vi "Nahum_spaceapps.vi"() -> ()   [LabVIEW 2013]
uses:
  <vilib>/Analysis/Matrix/Datatypes/RealMatrix.ctl
  <vilib>/Analysis/Matrix/Numeric/Conversions/Array To Matrix - RA2.vi
  <vilib>/Analysis/Matrix/NI_Matrix.lvlib
panel:
  out "Presion arterial":string
  out "RADIACIÓN AREA":string
  out "RC.PERSONA":string
  out "TEMP.AREA":string
  out "RADIACION EEI":string
  out "TEMP. PERSONA":string
  out "HUMEDAD AREA":string
  out "OXIGENO AREA":string
  out "VELOCIDAD EEI":string
  out "LATITUD EEI":string
  out "PRESIÓN AREA":string
  out "ILUMINACIÓN AREA":string
  out "ALTITUD EEI":string
  out "LONGITUD EEI":string
  out "GRAVEDAD AREA":string
  out "OXIGENO PERSONA":string
  out "ENERGIA":string
  out "GRAVEDAD AREA":dbl
  out "LATITUD EEI":dbl
  out "RADIACION AREA":dbl
  out "ILUMINACION AREA":dbl
  out "HUMEDAD AREA":dbl
  out "OXIGENO AREA":dbl
  out "PRESION AREA":dbl
  out "TEMP. AREA":dbl
  out "OXIGENO PERSONA":dbl
  out "RC. PERSONA":dbl
  out "PA.PERSONA":dbl
  out "TEMP.PERSONA":dbl
  out "LONGITUD EEI":dbl
  out "ALTITUD EEI":dbl
  out "VELOCIDAD EEI":dbl
  out "RADIACION EEI":dbl
  out "ENERGIA":dbl
  out "ENERGIA":T1
  out "ENERGIA":dbl[][](array[numeric])
  out "RADIACION EEI":T1
  out "RADIACION EEI":dbl[][](array[numeric])
  out "VELOCIDAD EEI":T1
  out "VELOCIDAD EEI":dbl[][](array[numeric])
  out "ALTITUD EEI":T1
  out "ALTITUD EEI":dbl[][](array[numeric])
  out "LONGITUD EEI":T1
  out "LONGITUD EEI":dbl[][](array[numeric])
  out "LATITUD EEI":T1
  out "LATITUD EEI":dbl[][](array[numeric])
  out "ILUMINACION AREA":T1
  out "ILUMINACION AREA":dbl[][](array[numeric])
  out "GRAVEDAD AREA":T1
  out "GRAVEDAD AREA":dbl[][](array[numeric])
  out "HUMEDAD AREA":T1
  out "HUMEDAD AREA":dbl[][](array[numeric])
  out "RADIACION AREA":T1
  out "RADIACION AREA":dbl[][](array[numeric])
  out "OXIGENO AREA":T1
  out "OXIGENO AREA":dbl[][](array[numeric])
  out "PRESION AREA":T1
  out "PRESION AREA":dbl[][](array[numeric])
  out "TEMP. AREA":T1
  out "TEMP. AREA":dbl[][](array[numeric])
  out "Oxigeno PERSONA":T1
  out "Oxigeno SANGRE PERSONA":dbl[][](array[numeric])
  out "RC. PERSONA":T1
  out "Ritmo Cardiaco":dbl[][](array[numeric])
  out "PA. PERSONA":T1
  out "PRESION ARTERIAL PERSONA":dbl[][](array[numeric])
  out "TEMP.PERSONA":T1
  out "TEMP.PERSONA":dbl[][](array[numeric])
  out "R10":dbl
  out "R9":dbl
  out "R8":dbl
  out "R7":dbl
  out "R6":dbl
  out "R5":dbl
  out "R4":dbl
  out "R3":dbl
  out "R2":dbl
  in  "stop":bool
  out "R1":dbl
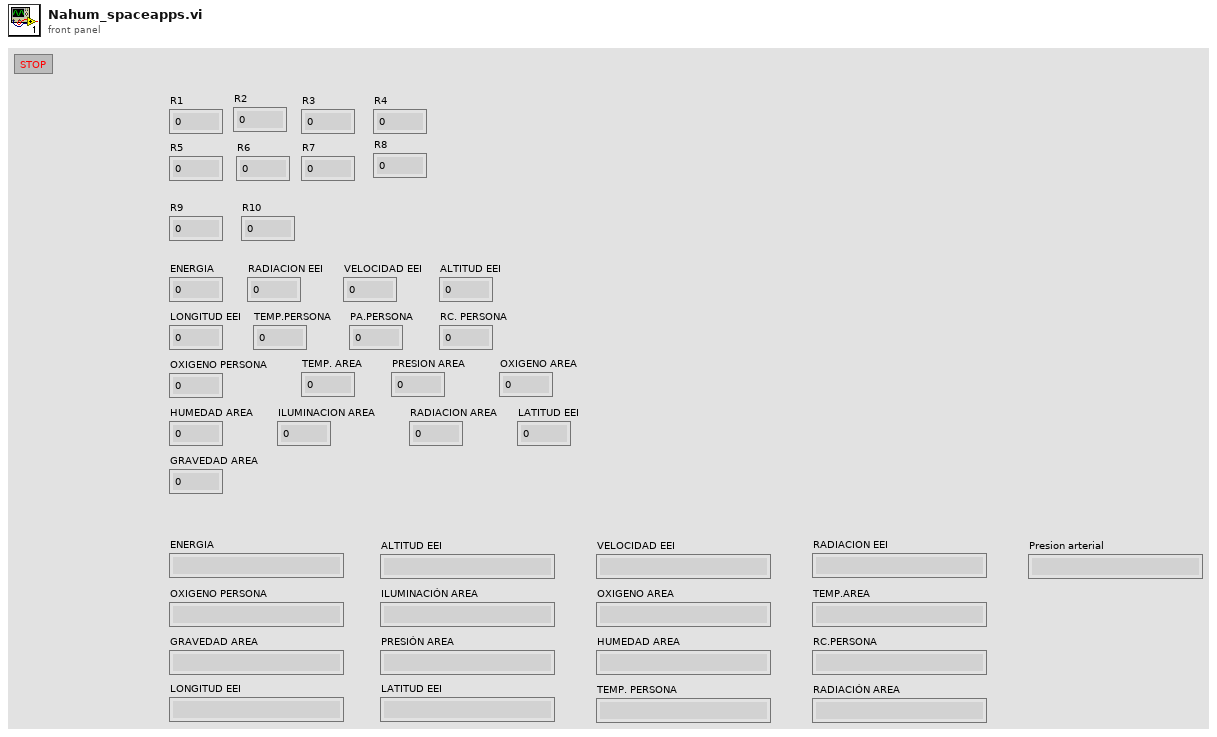
[diagram p1: front panel]
types:
  T1 = typedef "NI_Matrix.lvlib/RealMatrix.ctl" = dbl[][]
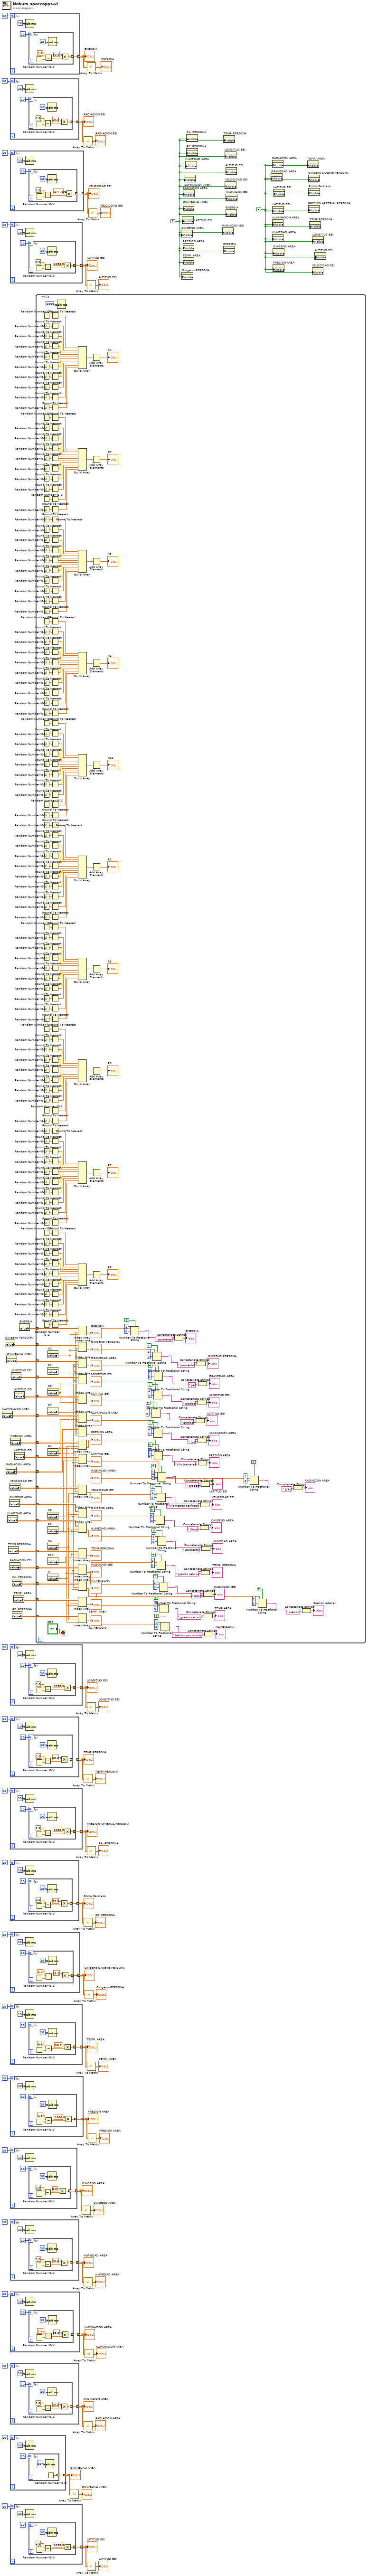
[diagram p0: block diagram]
diagram:
  w2 = FALSE
  w1 = FALSE
  n1 = property on="ILUMINACION AREA" class="Arr (strict)"() -> ("Value"=w6:T1)  [unwired: 2 in, 2 out]
  n2 = property on="Oxigeno PERSONA" class="Arr (strict)"() -> ("Value"=w11:T1)  [unwired: 2 in, 2 out]
  n3 = property on="RADIACION AREA" class="Arr (strict)"() -> ("Value"=w5:T1)  [unwired: 2 in, 2 out]
  n4 = property on="GRAVEDAD AREA" class="Arr (strict)"() -> ("Value"=w3:T1)  [unwired: 2 in, 2 out]
  n5 = property on="HUMEDAD AREA" class="Arr (strict)"() -> ("Value"=w7:T1)  [unwired: 2 in, 2 out]
  n6 = property on="TEMP.PERSONA" class="Arr (strict)"() -> ("Value"=w14:T1)  [unwired: 2 in, 2 out]
  n7 = property on="OXIGENO AREA" class="Arr (strict)"() -> ("Value"=w8:T1)  [unwired: 2 in, 2 out]
  n8 = property on="VELOCIDAD EEI" class="Arr (strict)"() -> ("Value"=w17:T1)  [unwired: 2 in, 2 out]
  n9 = property on="RADIACION EEI" class="Arr (strict)"() -> ("Value"=w18:T1)  [unwired: 2 in, 2 out]
  n10 = for {
    N: 10 -> [_]
    tunnel: [w73] -> w22 mode=indexing
    n11 = Wait (ms)(milliseconds to wait=u32 10) -> ()  [unwired: 1 out]
    n12 = for {
      N: 10 -> [_]
      tunnel: [w74] -> w73 mode=indexing
      n13 = Random Number (0-1)() -> (number: 0 to 1=w77:dbl)
      n14 = Subtract(x=1.8, y=w77) -> (x-y=w76:dbl)
      n15 = Wait (ms)(milliseconds to wait=u32 10) -> ()  [unwired: 1 out]
      n16 = Multiply(x=80.0, y=w76) -> (x*y=w74:dbl)
    }
  }
  "ENERGIA" <- w22
  n17 = for {
    N: 10 -> [_]
    tunnel: [w82] -> w25 mode=indexing
    n18 = Wait (ms)(milliseconds to wait=u32 10) -> ()  [unwired: 1 out]
    n19 = for {
      N: 10 -> [_]
      tunnel: [w83] -> w82 mode=indexing
      n20 = Random Number (0-1)() -> (number: 0 to 1=w86:dbl)
      n21 = Subtract(x=1.0, y=w86) -> (x-y=w85:dbl)
      n22 = Wait (ms)(milliseconds to wait=u32 10) -> ()  [unwired: 1 out]
      n23 = Multiply(x=10.0, y=w85) -> (x*y=w83:dbl)
    }
  }
  "RADIACION EEI" <- w25
  n24 = for {
    N: 10 -> [_]
    tunnel: [w91] -> w28 mode=indexing
    n25 = Wait (ms)(milliseconds to wait=u32 10) -> ()  [unwired: 1 out]
    n26 = for {
      N: 10 -> [_]
      tunnel: [w92] -> w91 mode=indexing
      n27 = Random Number (0-1)() -> (number: 0 to 1=w95:dbl)
      n28 = Subtract(x=2.0, y=w95) -> (x-y=w94:dbl)
      n29 = Wait (ms)(milliseconds to wait=u32 10) -> ()  [unwired: 1 out]
      n30 = Multiply(x=27743.0, y=w94) -> (x*y=w92:dbl)
    }
  }
  "VELOCIDAD EEI" <- w28
  n31 = for {
    N: 10 -> [_]
    tunnel: [w100] -> w31 mode=indexing
    n32 = Wait (ms)(milliseconds to wait=u32 10) -> ()  [unwired: 1 out]
    n33 = for {
      N: 10 -> [_]
      tunnel: [w101] -> w100 mode=indexing
      n34 = Random Number (0-1)() -> (number: 0 to 1=w104:dbl)
      n35 = Subtract(x=2.0, y=w104) -> (x-y=w103:dbl)
      n36 = Wait (ms)(milliseconds to wait=u32 10) -> ()  [unwired: 1 out]
      n37 = Multiply(x=1250.0, y=w103) -> (x*y=w101:dbl)
    }
  }
  "ALTITUD EEI" <- w31
  n38 = for {
    N: 10 -> [_]
    tunnel: [w109] -> w34 mode=indexing
    n39 = Wait (ms)(milliseconds to wait=u32 10) -> ()  [unwired: 1 out]
    n40 = for {
      N: 10 -> [_]
      tunnel: [w110] -> w109 mode=indexing
      n41 = Random Number (0-1)() -> (number: 0 to 1=w113:dbl)
      n42 = Subtract(x=2.0, y=w113) -> (x-y=w112:dbl)
      n43 = Wait (ms)(milliseconds to wait=u32 10) -> ()  [unwired: 1 out]
      n44 = Multiply(x=1250.0, y=w112) -> (x*y=w110:dbl)
    }
  }
  "LONGITUD EEI" <- w34
  n45 = for {
    N: 10 -> [_]
    tunnel: [w118] -> w70 mode=indexing
    n46 = Wait (ms)(milliseconds to wait=u32 10) -> ()  [unwired: 1 out]
    n47 = for {
      N: 10 -> [_]
      tunnel: [w119] -> w118 mode=indexing
      n48 = Random Number (0-1)() -> (number: 0 to 1=w122:dbl)
      n49 = Subtract(x=2.0, y=w122) -> (x-y=w121:dbl)
      n50 = Wait (ms)(milliseconds to wait=u32 10) -> ()  [unwired: 1 out]
      n51 = Multiply(x=29.0, y=w121) -> (x*y=w119:dbl)
    }
  }
  "TEMP.PERSONA" <- w70
  n52 = for {
    N: 10 -> [_]
    tunnel: [w127] -> w68 mode=indexing
    n53 = Wait (ms)(milliseconds to wait=u32 10) -> ()  [unwired: 1 out]
    n54 = for {
      N: 10 -> [_]
      tunnel: [w128] -> w127 mode=indexing
      n55 = Random Number (0-1)() -> (number: 0 to 1=w131:dbl)
      n56 = Subtract(x=2.0, y=w131) -> (x-y=w130:dbl)
      n57 = Wait (ms)(milliseconds to wait=u32 10) -> ()  [unwired: 1 out]
      n58 = Multiply(x=1250.0, y=w130) -> (x*y=w128:dbl)
    }
  }
  "PRESION ARTERIAL PERSONA" <- w68
  n59 = for {
    N: 10 -> [_]
    tunnel: [w136] -> w64 mode=indexing
    n60 = Wait (ms)(milliseconds to wait=u32 10) -> ()  [unwired: 1 out]
    n61 = for {
      N: 10 -> [_]
      tunnel: [w137] -> w136 mode=indexing
      n62 = Random Number (0-1)() -> (number: 0 to 1=w140:dbl)
      n63 = Subtract(x=2.0, y=w140) -> (x-y=w139:dbl)
      n64 = Wait (ms)(milliseconds to wait=u32 10) -> ()  [unwired: 1 out]
      n65 = Multiply(x=55.0, y=w139) -> (x*y=w137:dbl)
    }
  }
  "Ritmo Cardiaco" <- w64
  n66 = for {
    N: 10 -> [_]
    tunnel: [w145] -> w62 mode=indexing
    n67 = Wait (ms)(milliseconds to wait=u32 10) -> ()  [unwired: 1 out]
    n68 = for {
      N: 10 -> [_]
      tunnel: [w146] -> w145 mode=indexing
      n69 = Random Number (0-1)() -> (number: 0 to 1=w149:dbl)
      n70 = Subtract(x=1.4, y=w149) -> (x-y=w148:dbl)
      n71 = Wait (ms)(milliseconds to wait=u32 10) -> ()  [unwired: 1 out]
      n72 = Multiply(x=95.0, y=w148) -> (x*y=w146:dbl)
    }
  }
  "Oxigeno SANGRE PERSONA" <- w62
  n73 = for {
    N: 10 -> [_]
    tunnel: [w154] -> w58 mode=indexing
    n74 = Wait (ms)(milliseconds to wait=u32 10) -> ()  [unwired: 1 out]
    n75 = for {
      N: 10 -> [_]
      tunnel: [w155] -> w154 mode=indexing
      n76 = Random Number (0-1)() -> (number: 0 to 1=w158:dbl)
      n77 = Subtract(x=1.6, y=w158) -> (x-y=w157:dbl)
      n78 = Wait (ms)(milliseconds to wait=u32 10) -> ()  [unwired: 1 out]
      n79 = Multiply(x=26.5, y=w157) -> (x*y=w155:dbl)
    }
  }
  "TEMP. AREA" <- w58
  n80 = for {
    N: 10 -> [_]
    tunnel: [w163] -> w55 mode=indexing
    n81 = Wait (ms)(milliseconds to wait=u32 10) -> ()  [unwired: 1 out]
    n82 = for {
      N: 10 -> [_]
      tunnel: [w164] -> w163 mode=indexing
      n83 = Random Number (0-1)() -> (number: 0 to 1=w167:dbl)
      n84 = Subtract(x=1.5, y=w167) -> (x-y=w166:dbl)
      n85 = Wait (ms)(milliseconds to wait=u32 10) -> ()  [unwired: 1 out]
      n86 = Multiply(x=1000.0, y=w166) -> (x*y=w164:dbl)
    }
  }
  "PRESION AREA" <- w55
  n87 = for {
    N: 10 -> [_]
    tunnel: [w172] -> w52 mode=indexing
    n88 = Wait (ms)(milliseconds to wait=u32 10) -> ()  [unwired: 1 out]
    n89 = for {
      N: 10 -> [_]
      tunnel: [w173] -> w172 mode=indexing
      n90 = Random Number (0-1)() -> (number: 0 to 1=w176:dbl)
      n91 = Subtract(x=2.0, y=w176) -> (x-y=w175:dbl)
      n92 = Wait (ms)(milliseconds to wait=u32 10) -> ()  [unwired: 1 out]
      n93 = Multiply(x=6.0, y=w175) -> (x*y=w173:dbl)
    }
  }
  "OXIGENO AREA" <- w52
  n94 = for {
    N: 10 -> [_]
    tunnel: [w181] -> w46 mode=indexing
    n95 = Wait (ms)(milliseconds to wait=u32 10) -> ()  [unwired: 1 out]
    n96 = for {
      N: 10 -> [_]
      tunnel: [w182] -> w181 mode=indexing
      n97 = Random Number (0-1)() -> (number: 0 to 1=w185:dbl)
      n98 = Subtract(x=2.0, y=w185) -> (x-y=w184:dbl)
      n99 = Wait (ms)(milliseconds to wait=u32 10) -> ()  [unwired: 1 out]
      n100 = Multiply(x=40.0, y=w184) -> (x*y=w182:dbl)
    }
  }
  "HUMEDAD AREA" <- w46
  n101 = for {
    N: 10 -> [_]
    tunnel: [w190] -> w40 mode=indexing
    n102 = Wait (ms)(milliseconds to wait=u32 10) -> ()  [unwired: 1 out]
    n103 = for {
      N: 10 -> [_]
      tunnel: [w191] -> w190 mode=indexing
      n104 = Random Number (0-1)() -> (number: 0 to 1=w194:dbl)
      n105 = Subtract(x=1.4, y=w194) -> (x-y=w193:dbl)
      n106 = Wait (ms)(milliseconds to wait=u32 10) -> ()  [unwired: 1 out]
      n107 = Multiply(x=95.0, y=w193) -> (x*y=w191:dbl)
    }
  }
  "ILUMINACION AREA" <- w40
  n108 = for {
    N: 10 -> [_]
    tunnel: [w199] -> w49 mode=indexing
    n109 = Wait (ms)(milliseconds to wait=u32 10) -> ()  [unwired: 1 out]
    n110 = for {
      N: 10 -> [_]
      tunnel: [w200] -> w199 mode=indexing
      n111 = Random Number (0-1)() -> (number: 0 to 1=w203:dbl)
      n112 = Subtract(x=2.0, y=w203) -> (x-y=w202:dbl)
      n113 = Wait (ms)(milliseconds to wait=u32 10) -> ()  [unwired: 1 out]
      n114 = Multiply(x=10.0, y=w202) -> (x*y=w200:dbl)
    }
  }
  "RADIACION AREA" <- w49
  n115 = for {
    N: 10 -> [_]
    tunnel: [w208] -> w43 mode=indexing
    n116 = Wait (ms)(milliseconds to wait=u32 10) -> ()  [unwired: 1 out]
    n117 = for {
      N: 10 -> [_]
      tunnel: [w209] -> w208 mode=indexing
      n118 = Wait (ms)(milliseconds to wait=u32 10) -> ()  [unwired: 1 out]
      n119 = Random Number (0-1)() -> (number: 0 to 1=w209:dbl)
    }
  }
  "GRAVEDAD AREA" <- w43
  n120 = for {
    N: 10 -> [_]
    tunnel: [w213] -> w37 mode=indexing
    n121 = Wait (ms)(milliseconds to wait=u32 10) -> ()  [unwired: 1 out]
    n122 = for {
      N: 10 -> [_]
      tunnel: [w214] -> w213 mode=indexing
      n123 = Random Number (0-1)() -> (number: 0 to 1=w217:dbl)
      n124 = Subtract(x=2.0, y=w217) -> (x-y=w216:dbl)
      n125 = Wait (ms)(milliseconds to wait=u32 10) -> ()  [unwired: 1 out]
      n126 = Multiply(x=1250.0, y=w216) -> (x*y=w214:dbl)
    }
  }
  "LATITUD EEI" <- w37
  n127 = property on="PRESION AREA" class="Arr (strict)"() -> ("Value"=w9:T1)  [unwired: 2 in, 2 out]
  n128 = property on="LONGITUD EEI" class="Arr (strict)"() -> ("Value"=w15:T1)  [unwired: 2 in, 2 out]
  n129 = property on="PA. PERSONA" class="Arr (strict)"() -> ("Value"=w13:T1)  [unwired: 2 in, 2 out]
  n130 = property on="RC. PERSONA" class="Arr (strict)"() -> ("Value"=w12:T1)  [unwired: 2 in, 2 out]
  n131 = property on="TEMP. AREA" class="Arr (strict)"() -> ("Value"=w10:T1)  [unwired: 2 in, 2 out]
  n132 = property on="ALTITUD EEI" class="Arr (strict)"() -> ("Value"=w16:T1)  [unwired: 2 in, 2 out]
  n133 = property on="LATITUD EEI" class="Arr (strict)"() -> ("Value"=w4:T1)  [unwired: 2 in, 2 out]
  n134 = property on="ENERGIA" class="Arr (strict)"() -> ("Value"=w19:T1)  [unwired: 2 in, 2 out]
  n135 = while {
    tunnel: w19 -> [w365]
    tunnel: w18 -> [w364]
    tunnel: w17 -> [w363]
    tunnel: w16 -> [w362]
    tunnel: w15 -> [w361]
    tunnel: w14 -> [w360]
    tunnel: w13 -> [w359]
    tunnel: w12 -> [w358]
    tunnel: w11 -> [w357]
    tunnel: w10 -> [w356]
    tunnel: w9 -> [w355]
    tunnel: w8 -> [w354]
    tunnel: w7 -> [w353]
    tunnel: w6 -> [w352]
    tunnel: w5 -> [w351]
    tunnel: w4 -> [w350]
    tunnel: w3 -> [w349]
    stop <- "stop" stop-if-true
    n136 = Random Number (0-1)() -> (number: 0 to 1=w500:dbl)
    n137 = Random Number (0-1)() -> (number: 0 to 1=w501:dbl)
    n138 = Random Number (0-1)() -> (number: 0 to 1=w502:dbl)
    n139 = Random Number (0-1)() -> (number: 0 to 1=w503:dbl)
    n140 = Random Number (0-1)() -> (number: 0 to 1=w504:dbl)
    n141 = Random Number (0-1)() -> (number: 0 to 1=w505:dbl)
    n142 = Random Number (0-1)() -> (number: 0 to 1=w506:dbl)
    n143 = Random Number (0-1)() -> (number: 0 to 1=w507:dbl)
    n144 = Random Number (0-1)() -> (number: 0 to 1=w508:dbl)
    n145 = Random Number (0-1)() -> (number: 0 to 1=w509:dbl)
    n146 = Random Number (0-1)() -> (number: 0 to 1=w434:dbl)
    n147 = Random Number (0-1)() -> (number: 0 to 1=w435:dbl)
    n148 = Random Number (0-1)() -> (number: 0 to 1=w436:dbl)
    n149 = Random Number (0-1)() -> (number: 0 to 1=w437:dbl)
    n150 = Random Number (0-1)() -> (number: 0 to 1=w438:dbl)
    n151 = Random Number (0-1)() -> (number: 0 to 1=w439:dbl)
    n152 = Random Number (0-1)() -> (number: 0 to 1=w440:dbl)
    n153 = Random Number (0-1)() -> (number: 0 to 1=w441:dbl)
    n154 = Random Number (0-1)() -> (number: 0 to 1=w442:dbl)
    n155 = Random Number (0-1)() -> (number: 0 to 1=w443:dbl)
    n156 = Random Number (0-1)() -> (number: 0 to 1=w478:dbl)
    n157 = Random Number (0-1)() -> (number: 0 to 1=w479:dbl)
    n158 = Random Number (0-1)() -> (number: 0 to 1=w480:dbl)
    n159 = Random Number (0-1)() -> (number: 0 to 1=w481:dbl)
    n160 = Random Number (0-1)() -> (number: 0 to 1=w482:dbl)
    n161 = Random Number (0-1)() -> (number: 0 to 1=w483:dbl)
    n162 = Random Number (0-1)() -> (number: 0 to 1=w484:dbl)
    n163 = Random Number (0-1)() -> (number: 0 to 1=w485:dbl)
    n164 = Random Number (0-1)() -> (number: 0 to 1=w486:dbl)
    n165 = Random Number (0-1)() -> (number: 0 to 1=w487:dbl)
    n166 = Random Number (0-1)() -> (number: 0 to 1=w456:dbl)
    n167 = Random Number (0-1)() -> (number: 0 to 1=w457:dbl)
    n168 = Random Number (0-1)() -> (number: 0 to 1=w458:dbl)
    n169 = Random Number (0-1)() -> (number: 0 to 1=w459:dbl)
    n170 = Random Number (0-1)() -> (number: 0 to 1=w460:dbl)
    n171 = Random Number (0-1)() -> (number: 0 to 1=w461:dbl)
    n172 = Random Number (0-1)() -> (number: 0 to 1=w462:dbl)
    n173 = Random Number (0-1)() -> (number: 0 to 1=w463:dbl)
    n174 = Random Number (0-1)() -> (number: 0 to 1=w464:dbl)
    n175 = Random Number (0-1)() -> (number: 0 to 1=w465:dbl)
    n176 = Random Number (0-1)() -> (number: 0 to 1=w368:dbl)
    n177 = Random Number (0-1)() -> (number: 0 to 1=w369:dbl)
    n178 = Random Number (0-1)() -> (number: 0 to 1=w370:dbl)
    n179 = Random Number (0-1)() -> (number: 0 to 1=w371:dbl)
    n180 = Random Number (0-1)() -> (number: 0 to 1=w372:dbl)
    n181 = Random Number (0-1)() -> (number: 0 to 1=w373:dbl)
    n182 = Random Number (0-1)() -> (number: 0 to 1=w374:dbl)
    n183 = Random Number (0-1)() -> (number: 0 to 1=w375:dbl)
    n184 = Random Number (0-1)() -> (number: 0 to 1=w376:dbl)
    n185 = Random Number (0-1)() -> (number: 0 to 1=w377:dbl)
    n186 = Random Number (0-1)() -> (number: 0 to 1=w567:dbl)
    n187 = Random Number (0-1)() -> (number: 0 to 1=w568:dbl)
    n188 = Random Number (0-1)() -> (number: 0 to 1=w569:dbl)
    n189 = Random Number (0-1)() -> (number: 0 to 1=w570:dbl)
    n190 = Random Number (0-1)() -> (number: 0 to 1=w571:dbl)
    n191 = Random Number (0-1)() -> (number: 0 to 1=w572:dbl)
    n192 = Random Number (0-1)() -> (number: 0 to 1=w573:dbl)
    n193 = Random Number (0-1)() -> (number: 0 to 1=w574:dbl)
    n194 = Random Number (0-1)() -> (number: 0 to 1=w575:dbl)
    n195 = Random Number (0-1)() -> (number: 0 to 1=w576:dbl)
    n196 = Random Number (0-1)() -> (number: 0 to 1=w522:dbl)
    n197 = Random Number (0-1)() -> (number: 0 to 1=w523:dbl)
    n198 = Random Number (0-1)() -> (number: 0 to 1=w524:dbl)
    n199 = Random Number (0-1)() -> (number: 0 to 1=w525:dbl)
    n200 = Random Number (0-1)() -> (number: 0 to 1=w526:dbl)
    n201 = Random Number (0-1)() -> (number: 0 to 1=w527:dbl)
    n202 = Random Number (0-1)() -> (number: 0 to 1=w528:dbl)
    n203 = Random Number (0-1)() -> (number: 0 to 1=w529:dbl)
    n204 = Random Number (0-1)() -> (number: 0 to 1=w530:dbl)
    n205 = Random Number (0-1)() -> (number: 0 to 1=w531:dbl)
    n206 = Random Number (0-1)() -> (number: 0 to 1=w390:dbl)
    n207 = Random Number (0-1)() -> (number: 0 to 1=w391:dbl)
    n208 = Random Number (0-1)() -> (number: 0 to 1=w392:dbl)
    n209 = Random Number (0-1)() -> (number: 0 to 1=w393:dbl)
    n210 = Random Number (0-1)() -> (number: 0 to 1=w394:dbl)
    n211 = Random Number (0-1)() -> (number: 0 to 1=w395:dbl)
    n212 = Random Number (0-1)() -> (number: 0 to 1=w396:dbl)
    n213 = Random Number (0-1)() -> (number: 0 to 1=w397:dbl)
    n214 = Random Number (0-1)() -> (number: 0 to 1=w398:dbl)
    n215 = Random Number (0-1)() -> (number: 0 to 1=w399:dbl)
    n216 = Random Number (0-1)() -> (number: 0 to 1=w544:dbl)
    n217 = Random Number (0-1)() -> (number: 0 to 1=w545:dbl)
    n218 = Random Number (0-1)() -> (number: 0 to 1=w546:dbl)
    n219 = Random Number (0-1)() -> (number: 0 to 1=w547:dbl)
    n220 = Random Number (0-1)() -> (number: 0 to 1=w548:dbl)
    n221 = Random Number (0-1)() -> (number: 0 to 1=w549:dbl)
    n222 = Random Number (0-1)() -> (number: 0 to 1=w550:dbl)
    n223 = Random Number (0-1)() -> (number: 0 to 1=w551:dbl)
    n224 = Random Number (0-1)() -> (number: 0 to 1=w552:dbl)
    n225 = Random Number (0-1)() -> (number: 0 to 1=w553:dbl)
    n226 = Random Number (0-1)() -> (number: 0 to 1=w412:dbl)
    n227 = Random Number (0-1)() -> (number: 0 to 1=w413:dbl)
    n228 = Random Number (0-1)() -> (number: 0 to 1=w414:dbl)
    n229 = Random Number (0-1)() -> (number: 0 to 1=w415:dbl)
    n230 = Random Number (0-1)() -> (number: 0 to 1=w416:dbl)
    n231 = Random Number (0-1)() -> (number: 0 to 1=w417:dbl)
    n232 = Random Number (0-1)() -> (number: 0 to 1=w418:dbl)
    n233 = Random Number (0-1)() -> (number: 0 to 1=w419:dbl)
    n234 = Random Number (0-1)() -> (number: 0 to 1=w420:dbl)
    n235 = Random Number (0-1)() -> (number: 0 to 1=w421:dbl)
    n236 = property on="R2" class="DigNum (strict)"() -> ("Value"=w346:dbl)  [unwired: 2 in, 2 out]
    n237 = property on="R1" class="DigNum (strict)"() -> ("Value"=w342:dbl)  [unwired: 2 in, 2 out]
    n238 = property on="R8" class="DigNum (strict)"() -> ("Value"=w347:dbl)  [unwired: 2 in, 2 out]
    n239 = property on="R7" class="DigNum (strict)"() -> ("Value"=w343:dbl)  [unwired: 2 in, 2 out]
    n240 = property on="R5" class="DigNum (strict)"() -> ("Value"=w344:dbl)  [unwired: 2 in, 2 out]
    n241 = property on="R3" class="DigNum (strict)"() -> ("Value"=w339:dbl)  [unwired: 2 in, 2 out]
    n242 = property on="R9" class="DigNum (strict)"() -> ("Value"=w341:dbl)  [unwired: 2 in, 2 out]
    n243 = property on="R6" class="DigNum (strict)"() -> ("Value"=w340:dbl)  [unwired: 2 in, 2 out]
    n244 = property on="R10" class="DigNum (strict)"() -> ("Value"=w348:dbl)  [unwired: 2 in, 2 out]
    n245 = property on="R4" class="DigNum (strict)"() -> ("Value"=w345:dbl)  [unwired: 2 in, 2 out]
    n246 = Round To Nearest(number=w500) -> (nearest integer value=w510:dbl)
    n247 = Round To Nearest(number=w501) -> (nearest integer value=w511:dbl)
    n248 = Round To Nearest(number=w502) -> (nearest integer value=w512:dbl)
    n249 = Round To Nearest(number=w503) -> (nearest integer value=w513:dbl)
    n250 = Round To Nearest(number=w504) -> (nearest integer value=w514:dbl)
    n251 = Round To Nearest(number=w505) -> (nearest integer value=w515:dbl)
    n252 = Round To Nearest(number=w506) -> (nearest integer value=w516:dbl)
    n253 = Round To Nearest(number=w507) -> (nearest integer value=w517:dbl)
    n254 = Round To Nearest(number=w508) -> (nearest integer value=w518:dbl)
    n255 = Round To Nearest(number=w509) -> (nearest integer value=w519:dbl)
    n256 = Round To Nearest(number=w434) -> (nearest integer value=w444:dbl)
    n257 = Round To Nearest(number=w435) -> (nearest integer value=w445:dbl)
    n258 = Round To Nearest(number=w436) -> (nearest integer value=w446:dbl)
    n259 = Round To Nearest(number=w437) -> (nearest integer value=w447:dbl)
    n260 = Round To Nearest(number=w438) -> (nearest integer value=w448:dbl)
    n261 = Round To Nearest(number=w439) -> (nearest integer value=w449:dbl)
    n262 = Round To Nearest(number=w440) -> (nearest integer value=w450:dbl)
    n263 = Round To Nearest(number=w441) -> (nearest integer value=w451:dbl)
    n264 = Round To Nearest(number=w442) -> (nearest integer value=w452:dbl)
    n265 = Round To Nearest(number=w443) -> (nearest integer value=w453:dbl)
    n266 = Round To Nearest(number=w478) -> (nearest integer value=w488:dbl)
    n267 = Round To Nearest(number=w479) -> (nearest integer value=w489:dbl)
    n268 = Round To Nearest(number=w480) -> (nearest integer value=w490:dbl)
    n269 = Round To Nearest(number=w481) -> (nearest integer value=w491:dbl)
    n270 = Round To Nearest(number=w482) -> (nearest integer value=w492:dbl)
    n271 = Round To Nearest(number=w483) -> (nearest integer value=w493:dbl)
    n272 = Round To Nearest(number=w484) -> (nearest integer value=w494:dbl)
    n273 = Round To Nearest(number=w485) -> (nearest integer value=w495:dbl)
    n274 = Round To Nearest(number=w486) -> (nearest integer value=w496:dbl)
    n275 = Round To Nearest(number=w487) -> (nearest integer value=w497:dbl)
    n276 = Round To Nearest(number=w456) -> (nearest integer value=w466:dbl)
    n277 = Round To Nearest(number=w457) -> (nearest integer value=w467:dbl)
    n278 = Round To Nearest(number=w458) -> (nearest integer value=w468:dbl)
    n279 = Round To Nearest(number=w459) -> (nearest integer value=w469:dbl)
    n280 = Round To Nearest(number=w460) -> (nearest integer value=w470:dbl)
    n281 = Round To Nearest(number=w461) -> (nearest integer value=w471:dbl)
    n282 = Round To Nearest(number=w462) -> (nearest integer value=w472:dbl)
    n283 = Round To Nearest(number=w463) -> (nearest integer value=w473:dbl)
    n284 = Round To Nearest(number=w464) -> (nearest integer value=w474:dbl)
    n285 = Round To Nearest(number=w465) -> (nearest integer value=w475:dbl)
    n286 = Round To Nearest(number=w368) -> (nearest integer value=w378:dbl)
    n287 = Round To Nearest(number=w369) -> (nearest integer value=w379:dbl)
    n288 = Round To Nearest(number=w370) -> (nearest integer value=w380:dbl)
    n289 = Round To Nearest(number=w371) -> (nearest integer value=w381:dbl)
    n290 = Round To Nearest(number=w372) -> (nearest integer value=w382:dbl)
    n291 = Round To Nearest(number=w373) -> (nearest integer value=w383:dbl)
    n292 = Round To Nearest(number=w374) -> (nearest integer value=w384:dbl)
    n293 = Round To Nearest(number=w375) -> (nearest integer value=w385:dbl)
    n294 = Round To Nearest(number=w376) -> (nearest integer value=w386:dbl)
    n295 = Round To Nearest(number=w377) -> (nearest integer value=w387:dbl)
    n296 = Round To Nearest(number=w567) -> (nearest integer value=w577:dbl)
    n297 = Round To Nearest(number=w568) -> (nearest integer value=w578:dbl)
    n298 = Round To Nearest(number=w569) -> (nearest integer value=w579:dbl)
    n299 = Round To Nearest(number=w570) -> (nearest integer value=w580:dbl)
    n300 = Round To Nearest(number=w571) -> (nearest integer value=w581:dbl)
    n301 = Round To Nearest(number=w572) -> (nearest integer value=w582:dbl)
    n302 = Round To Nearest(number=w573) -> (nearest integer value=w583:dbl)
    n303 = Round To Nearest(number=w574) -> (nearest integer value=w584:dbl)
    n304 = Round To Nearest(number=w575) -> (nearest integer value=w585:dbl)
    n305 = Round To Nearest(number=w576) -> (nearest integer value=w586:dbl)
    n306 = Round To Nearest(number=w522) -> (nearest integer value=w532:dbl)
    n307 = Round To Nearest(number=w523) -> (nearest integer value=w533:dbl)
    n308 = Round To Nearest(number=w524) -> (nearest integer value=w534:dbl)
    n309 = Round To Nearest(number=w525) -> (nearest integer value=w535:dbl)
    n310 = Round To Nearest(number=w526) -> (nearest integer value=w536:dbl)
    n311 = Round To Nearest(number=w527) -> (nearest integer value=w537:dbl)
    n312 = Round To Nearest(number=w528) -> (nearest integer value=w538:dbl)
    n313 = Round To Nearest(number=w529) -> (nearest integer value=w539:dbl)
    n314 = Round To Nearest(number=w530) -> (nearest integer value=w540:dbl)
    n315 = Round To Nearest(number=w531) -> (nearest integer value=w541:dbl)
    n316 = Round To Nearest(number=w390) -> (nearest integer value=w400:dbl)
    n317 = Round To Nearest(number=w391) -> (nearest integer value=w401:dbl)
    n318 = Round To Nearest(number=w392) -> (nearest integer value=w402:dbl)
    n319 = Round To Nearest(number=w393) -> (nearest integer value=w403:dbl)
    n320 = Round To Nearest(number=w394) -> (nearest integer value=w404:dbl)
    n321 = Round To Nearest(number=w395) -> (nearest integer value=w405:dbl)
    n322 = Round To Nearest(number=w396) -> (nearest integer value=w406:dbl)
    n323 = Round To Nearest(number=w397) -> (nearest integer value=w407:dbl)
    n324 = Round To Nearest(number=w398) -> (nearest integer value=w408:dbl)
    n325 = Round To Nearest(number=w399) -> (nearest integer value=w409:dbl)
    n326 = Round To Nearest(number=w544) -> (nearest integer value=w554:dbl)
    n327 = Round To Nearest(number=w545) -> (nearest integer value=w555:dbl)
    n328 = Round To Nearest(number=w546) -> (nearest integer value=w556:dbl)
    n329 = Round To Nearest(number=w547) -> (nearest integer value=w557:dbl)
    n330 = Round To Nearest(number=w548) -> (nearest integer value=w558:dbl)
    n331 = Round To Nearest(number=w549) -> (nearest integer value=w559:dbl)
    n332 = Round To Nearest(number=w550) -> (nearest integer value=w560:dbl)
    n333 = Round To Nearest(number=w551) -> (nearest integer value=w561:dbl)
    n334 = Round To Nearest(number=w552) -> (nearest integer value=w562:dbl)
    n335 = Round To Nearest(number=w553) -> (nearest integer value=w563:dbl)
    n336 = Round To Nearest(number=w412) -> (nearest integer value=w422:dbl)
    n337 = Round To Nearest(number=w413) -> (nearest integer value=w423:dbl)
    n338 = Round To Nearest(number=w414) -> (nearest integer value=w424:dbl)
    n339 = Round To Nearest(number=w415) -> (nearest integer value=w425:dbl)
    n340 = Round To Nearest(number=w416) -> (nearest integer value=w426:dbl)
    n341 = Round To Nearest(number=w417) -> (nearest integer value=w427:dbl)
    n342 = Round To Nearest(number=w418) -> (nearest integer value=w428:dbl)
    n343 = Round To Nearest(number=w419) -> (nearest integer value=w429:dbl)
    n344 = Round To Nearest(number=w420) -> (nearest integer value=w430:dbl)
    n345 = Round To Nearest(number=w421) -> (nearest integer value=w431:dbl)
    n346 = Wait (ms)(milliseconds to wait=u32 2000) -> ()  [unwired: 1 out]
    n347 = Build Array(w510, w511, w512, w513, w514, w515, w516, w517, w518, w519) -> (w520:dbl[])
    n348 = Build Array(w444, w445, w446, w447, w448, w449, w450, w451, w452, w453) -> (w454:dbl[])
    n349 = Build Array(w488, w489, w490, w491, w492, w493, w494, w495, w496, w497) -> (w498:dbl[])
    n350 = Build Array(w466, w467, w468, w469, w470, w471, w472, w473, w474, w475) -> (w476:dbl[])
    n351 = Build Array(w378, w379, w380, w381, w382, w383, w384, w385, w386, w387) -> (w388:dbl[])
    n352 = Build Array(w577, w578, w579, w580, w581, w582, w583, w584, w585, w586) -> (w587:dbl[])
    n353 = Build Array(w532, w533, w534, w535, w536, w537, w538, w539, w540, w541) -> (w542:dbl[])
    n354 = Build Array(w400, w401, w402, w403, w404, w405, w406, w407, w408, w409) -> (w410:dbl[])
    n355 = Build Array(w554, w555, w556, w557, w558, w559, w560, w561, w562, w563) -> (w564:dbl[])
    n356 = Build Array(w422, w423, w424, w425, w426, w427, w428, w429, w430, w431) -> (w432:dbl[])
    n357 = Index Array(array=w365, index (row)=w342, index (col)=w346) -> (element=w338:dbl)
    "ENERGIA" <- w338
    n358 = Index Array(array=w357, index (row)=w343, index (col)=w346) -> (element=w325:dbl)
    "OXIGENO PERSONA" <- w325
    n359 = Index Array(array=w349, index (row)=w339, index (col)=w342) -> (element=w318:dbl)
    "GRAVEDAD AREA" <- w318
    n360 = Index Array(array=w361, index (row)=w342, index (col)=w347) -> (element=w311:dbl)
    "LONGITUD EEI" <- w311
    n361 = Index Array(array=w362, index (row)=w343, index (col)=w347) -> (element=w304:dbl)
    "ALTITUD EEI" <- w304
    n362 = Index Array(array=w352, index (row)=w344, index (col)=w343) -> (element=w297:dbl)
    "ILUMINACION AREA" <- w297
    n363 = Index Array(array=w351, index (row)=w343, index (col)=w342) -> (element=w227:dbl)
    "RADIACION AREA" <- w227
    n364 = Index Array(array=w355, index (row)=w345, index (col)=w344) -> (element=w290:dbl)
    "PRESION AREA" <- w290
    n365 = Index Array(array=w350, index (row)=w341, index (col)=w339) -> (element=w283:dbl)
    "LATITUD EEI" <- w283
    n366 = Index Array(array=w363, index (row)=w344, index (col)=w340) -> (element=w276:dbl)
    "VELOCIDAD EEI" <- w276
    n367 = Index Array(array=w354, index (row)=w340, index (col)=w339) -> (element=w269:dbl)
    "OXIGENO AREA" <- w269
    n368 = Index Array(array=w353, index (row)=w340, index (col)=w341) -> (element=w262:dbl)
    "HUMEDAD AREA" <- w262
    n369 = Index Array(array=w360, index (row)=w341, index (col)=w348) -> (element=w255:dbl)
    "TEMP.PERSONA" <- w255
    n370 = Index Array(array=w364, index (row)=w339, index (col)=w345) -> (element=w248:dbl)
    "RADIACION EEI" <- w248
    n371 = Index Array(array=w359, index (row)=w339, index (col)=w341) -> (element=w220:dbl)
    "PA.PERSONA" <- w220
    n372 = Index Array(array=w356, index (row)=w346, index (col)=w340) -> (element=w241:dbl)
    "TEMP. AREA" <- w241
    n373 = Index Array(array=w358, index (row)=w340, index (col)=w345) -> (element=w234:dbl)
    "RC. PERSONA" <- w234
    n374 = Add Array Elements(numeric array=w520) -> (sum=→"R4":dbl)
    n375 = Add Array Elements(numeric array=w454) -> (sum=→"R7":dbl)
    n376 = Add Array Elements(numeric array=w498) -> (sum=→"R5":dbl)
    n377 = Add Array Elements(numeric array=w476) -> (sum=→"R6":dbl)
    n378 = Add Array Elements(numeric array=w388) -> (sum=→"R10":dbl)
    n379 = Add Array Elements(numeric array=w587) -> (sum=→"R1":dbl)
    n380 = Add Array Elements(numeric array=w542) -> (sum=→"R3":dbl)
    n381 = Add Array Elements(numeric array=w410) -> (sum=→"R9":dbl)
    n382 = Add Array Elements(numeric array=w564) -> (sum=→"R2":dbl)
    n383 = Add Array Elements(numeric array=w432) -> (sum=→"R8":dbl)
    n384 = Number To Fractional String(use system decimal point (T)=TRUE, number=w338, width (-)=i16 0, precision (6)=i16 1) -> (F-format string=w333:string)
    n385 = Number To Fractional String(use system decimal point (T)=TRUE, number=w304, width (-)=i16 0, precision (6)=i16 1) -> (F-format string=w306:string)
    n386 = Number To Fractional String(use system decimal point (T)=TRUE, number=w325, width (-)=i16 0, precision (6)=i16 1) -> (F-format string=w327:string)
    n387 = Number To Fractional String(use system decimal point (T)=TRUE, number=w311, width (-)=i16 0, precision (6)=i16 1) -> (F-format string=w313:string)
    n388 = Number To Fractional String(use system decimal point (T)=TRUE, number=w297, width (-)=i16 0, precision (6)=i16 1) -> (F-format string=w299:string)
    n389 = Number To Fractional String(use system decimal point (T)=TRUE, number=w318, width (-)=i16 0, precision (6)=i16 1) -> (F-format string=w320:string)
    n390 = Number To Fractional String(use system decimal point (T)=TRUE, number=w290, width (-)=i16 0, precision (6)=i16 1) -> (F-format string=w292:string)
    n391 = Number To Fractional String(use system decimal point (T)=TRUE, number=w269, width (-)=i16 0, precision (6)=i16 1) -> (F-format string=w271:string)
    n392 = Number To Fractional String(use system decimal point (T)=TRUE, number=w276, width (-)=i16 0, precision (6)=i16 1) -> (F-format string=w278:string)
    n393 = Number To Fractional String(use system decimal point (T)=TRUE, number=w255, width (-)=i16 0, precision (6)=i16 1) -> (F-format string=w257:string)
    n394 = Number To Fractional String(use system decimal point (T)=TRUE, number=w283, width (-)=i16 0, precision (6)=i16 1) -> (F-format string=w285:string)
    n395 = Number To Fractional String(use system decimal point (T)=TRUE, number=w262, width (-)=i16 0, precision (6)=i16 1) -> (F-format string=w264:string)
    n396 = Number To Fractional String(use system decimal point (T)=TRUE, number=w248, width (-)=i16 0, precision (6)=i16 1) -> (F-format string=w250:string)
    n397 = Number To Fractional String(use system decimal point (T)=TRUE, number=w241, width (-)=i16 0, precision (6)=i16 1) -> (F-format string=w243:string)
    n398 = Number To Fractional String(use system decimal point (T)=TRUE, number=w234, width (-)=i16 0, precision (6)=i16 1) -> (F-format string=w236:string)
    n399 = Concatenate Strings(w333, " porciento" ("string")) -> (→"ENERGIA":string)
    n400 = Concatenate Strings(w306, " grados" ("string")) -> (→"ALTITUD EEI":string)
    n401 = Concatenate Strings(w327, " porciento" ("string")) -> (→"OXIGENO PERSONA":string)
    n402 = Concatenate Strings(w313, " grados" ("string")) -> (→"LONGITUD EEI":string)
    n403 = Concatenate Strings(w299, " lux" ("string")) -> (→"ILUMINACIÓN AREA":string)
    n404 = Concatenate Strings(w320, " jes" ("string")) -> (→"GRAVEDAD AREA":string)
    n405 = Concatenate Strings(w292, " kilo pascales" ("string")) -> (→"PRESIÓN AREA":string)
    n406 = Concatenate Strings(w271, " litros" ("string")) -> (→"OXIGENO AREA":string)
    n407 = Concatenate Strings(w278, " kilometros por hora" ("string")) -> (→"VELOCIDAD EEI":string)
    n408 = Concatenate Strings(w257, " grados celcius" ("string")) -> (→"TEMP. PERSONA":string)
    n409 = Concatenate Strings(w285, " grados" ("string")) -> (→"LATITUD EEI":string)
    n410 = Concatenate Strings(w264, " porciento" ("string")) -> (→"HUMEDAD AREA":string)
    n411 = Concatenate Strings(w250, " gray" ("string")) -> (→"RADIACION EEI":string)
    n412 = Concatenate Strings(w243, " grados celcius" ("string")) -> (→"TEMP.AREA":string)
    n413 = Concatenate Strings(w236, " latidos por minuto" ("string")) -> (→"RC.PERSONA":string)
    n414 = Number To Fractional String(use system decimal point (T)=TRUE, number=w227, width (-)=i16 0, precision (6)=i16 1) -> (F-format string=w230:string)
    n415 = Number To Fractional String(use system decimal point (T)=TRUE, number=w220, width (-)=i16 0, precision (6)=i16 1) -> (F-format string=w223:string)
    n416 = Concatenate Strings(w230, " gray" ("string")) -> (→"RADIACIÓN AREA":string)
    n417 = Concatenate Strings(w223, " presion" ("string")) -> (→"Presion arterial":string)
  }
  n418 = call-poly <vilib>:"Array To Matrix.vi"("Real 2D Array"=w43) -> ("Real Matrix"=→"GRAVEDAD AREA":T1)
  n419 = call-poly <vilib>:"Array To Matrix.vi"("Real 2D Array"=w52) -> ("Real Matrix"=→"OXIGENO AREA":T1)
  n420 = call-poly <vilib>:"Array To Matrix.vi"("Real 2D Array"=w25) -> ("Real Matrix"=→"RADIACION EEI":T1)
  n421 = call-poly <vilib>:"Array To Matrix.vi"("Real 2D Array"=w70) -> ("Real Matrix"=→"TEMP.PERSONA":T1)
  n422 = call-poly <vilib>:"Array To Matrix.vi"("Real 2D Array"=w64) -> ("Real Matrix"=→"RC. PERSONA":T1)
  n423 = call-poly <vilib>:"Array To Matrix.vi"("Real 2D Array"=w46) -> ("Real Matrix"=→"HUMEDAD AREA":T1)
  n424 = call-poly <vilib>:"Array To Matrix.vi"("Real 2D Array"=w49) -> ("Real Matrix"=→"RADIACION AREA":T1)
  n425 = call-poly <vilib>:"Array To Matrix.vi"("Real 2D Array"=w62) -> ("Real Matrix"=→"Oxigeno PERSONA":T1)
  n426 = call-poly <vilib>:"Array To Matrix.vi"("Real 2D Array"=w40) -> ("Real Matrix"=→"ILUMINACION AREA":T1)
  n427 = call-poly <vilib>:"Array To Matrix.vi"("Real 2D Array"=w22) -> ("Real Matrix"=→"ENERGIA":T1)
  n428 = call-poly <vilib>:"Array To Matrix.vi"("Real 2D Array"=w31) -> ("Real Matrix"=→"ALTITUD EEI":T1)
  n429 = call-poly <vilib>:"Array To Matrix.vi"("Real 2D Array"=w34) -> ("Real Matrix"=→"LONGITUD EEI":T1)
  n430 = call-poly <vilib>:"Array To Matrix.vi"("Real 2D Array"=w68) -> ("Real Matrix"=→"PA. PERSONA":T1)
  n431 = call-poly <vilib>:"Array To Matrix.vi"("Real 2D Array"=w58) -> ("Real Matrix"=→"TEMP. AREA":T1)
  n432 = call-poly <vilib>:"Array To Matrix.vi"("Real 2D Array"=w37) -> ("Real Matrix"=→"LATITUD EEI":T1)
  n433 = call-poly <vilib>:"Array To Matrix.vi"("Real 2D Array"=w55) -> ("Real Matrix"=→"PRESION AREA":T1)
  n434 = call-poly <vilib>:"Array To Matrix.vi"("Real 2D Array"=w28) -> ("Real Matrix"=→"VELOCIDAD EEI":T1)
  n435 = property on="OXIGENO AREA" class="Arr (strict)"("Visible"=w1) -> ()  [unwired: 2 in, 2 out]
  n436 = property on="Oxigeno PERSONA" class="Arr (strict)"("Visible"=w1) -> ()  [unwired: 2 in, 2 out]
  n437 = property on="LATITUD EEI" class="Arr (strict)"("Visible"=w1) -> ()  [unwired: 2 in, 2 out]
  n438 = property on="GRAVEDAD AREA" class="Arr (strict)"("Visible"=w1) -> ()  [unwired: 2 in, 2 out]
  n439 = property on="PRESION AREA" class="Arr (strict)"("Visible"=w1) -> ()  [unwired: 2 in, 2 out]
  n440 = property on="TEMP. AREA" class="Arr (strict)"("Visible"=w1) -> ()  [unwired: 2 in, 2 out]
  n441 = property on="RADIACION AREA" class="Arr (strict)"("Visible"=w1) -> ()  [unwired: 2 in, 2 out]
  n442 = property on="ILUMINACION AREA" class="Arr (strict)"("Visible"=w1) -> ()  [unwired: 2 in, 2 out]
  n443 = property on="HUMEDAD AREA" class="Arr (strict)"("Visible"=w1) -> ()  [unwired: 2 in, 2 out]
  n444 = property on="PA. PERSONA" class="Arr (strict)"("Visible"=w1) -> ()  [unwired: 2 in, 2 out]
  n445 = property on="RC. PERSONA" class="Arr (strict)"("Visible"=w1) -> ()  [unwired: 2 in, 2 out]
  n446 = property on="RADIACION EEI" class="Arr (strict)"("Visible"=w1) -> ()  [unwired: 2 in, 2 out]
  n447 = property on="ENERGIA" class="Arr (strict)"("Visible"=w1) -> ()  [unwired: 2 in, 2 out]
  n448 = property on="TEMP.PERSONA" class="Arr (strict)"("Visible"=w1) -> ()  [unwired: 2 in, 2 out]
  n449 = property on="LONGITUD EEI" class="Arr (strict)"("Visible"=w1) -> ()  [unwired: 2 in, 2 out]
  n450 = property on="VELOCIDAD EEI" class="Arr (strict)"("Visible"=w1) -> ()  [unwired: 2 in, 2 out]
  n451 = property on="ALTITUD EEI" class="Arr (strict)"("Visible"=w1) -> ()  [unwired: 2 in, 2 out]
  n452 = property on="ENERGIA" class="Arr (strict)"("Visible"=w1) -> ()  [unwired: 2 in, 2 out]
  n453 = property on="RADIACION EEI" class="Arr (strict)"("Visible"=w1) -> ()  [unwired: 2 in, 2 out]
  n454 = property on="GRAVEDAD AREA" class="Arr (strict)"("Visible"=w2) -> ()  [unwired: 2 in, 2 out]
  n455 = property on="RADIACION AREA" class="Arr (strict)"("Visible"=w2) -> ()  [unwired: 2 in, 2 out]
  n456 = property on="ILUMINACION AREA" class="Arr (strict)"("Visible"=w2) -> ()  [unwired: 2 in, 2 out]
  n457 = property on="HUMEDAD AREA" class="Arr (strict)"("Visible"=w2) -> ()  [unwired: 2 in, 2 out]
  n458 = property on="LATITUD EEI" class="Arr (strict)"("Visible"=w2) -> ()  [unwired: 2 in, 2 out]
  n459 = property on="OXIGENO AREA" class="Arr (strict)"("Visible"=w2) -> ()  [unwired: 2 in, 2 out]
  n460 = property on="PRESION AREA" class="Arr (strict)"("Visible"=w2) -> ()  [unwired: 2 in, 2 out]
  n461 = property on="LATITUD EEI" class="Arr (strict)"("Visible"=w2) -> ()  [unwired: 2 in, 2 out]
  n462 = property on="TEMP. AREA" class="Arr (strict)"("Visible"=w2) -> ()  [unwired: 2 in, 2 out]
  n463 = property on="Oxigeno SANGRE PERSONA" class="Arr (strict)"("Visible"=w2) -> ()  [unwired: 2 in, 2 out]
  n464 = property on="PRESION ARTERIAL PERSONA" class="Arr (strict)"("Visible"=w2) -> ()  [unwired: 2 in, 2 out]
  n465 = property on="Ritmo Cardiaco" class="Arr (strict)"("Visible"=w2) -> ()  [unwired: 2 in, 2 out]
  n466 = property on="TEMP.PERSONA" class="Arr (strict)"("Visible"=w2) -> ()  [unwired: 2 in, 2 out]
  n467 = property on="VELOCIDAD EEI" class="Arr (strict)"("Visible"=w2) -> ()  [unwired: 2 in, 2 out]
  n468 = property on="LONGITUD EEI" class="Arr (strict)"("Visible"=w2) -> ()  [unwired: 2 in, 2 out]
  n469 = property on="ALTITUD EEI" class="Arr (strict)"("Visible"=w2) -> ()  [unwired: 2 in, 2 out]
